vi "Problem 12 - Highly divisible triangular number.vi"(8 "error in (no error)":errorcluster) -> (0 "error out":errorcluster, 3 "Answer":u64)   [LabVIEW 2021, in "Project Euler.lvlib"]
uses:
  Project Euler.lvlib
  Utilities/Named Timers/Named Timers.lvlib
  Utilities/Numeric Utilities/Numeric Utilities.lvlib
panel:
  out "Triangular numbers":i32[](array[numeric])
  out "index of max no. of divisors":i32
  out "iteration execution time vs. iteration":u32[](graph)
  out "iteration execution time (ms)":u32
  in  "Dev: Stop early":bool
  out "max no. of divisors":i32
  in  "min requested no of divisors":i32=500
  in  "n = generate this many terms":u32=100
  out "Loop iteration":i32
  out "Total execution time (ms)":u32
  # "Development\ncontrols/indicators useful for development and testing, but which are not outputs of the VI"
  # "Input\nInputs to the VI"
  # "Output\nOutputs of the VI"
  # "Description\n\nBlank VI with error handling case. \n\nSummarize the use of this VI in this space."
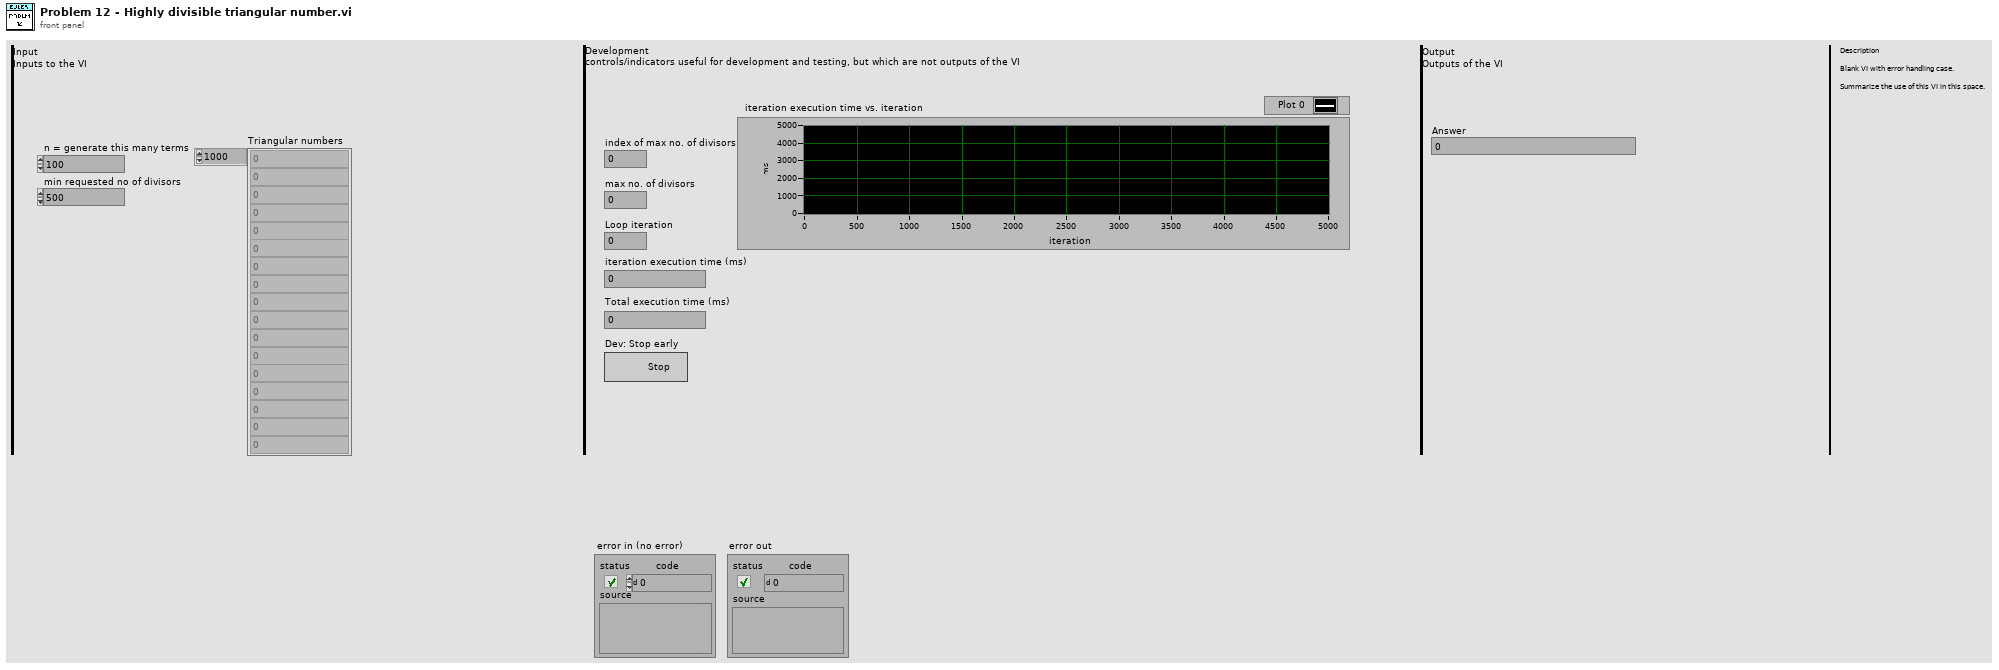
[diagram p1: front panel]
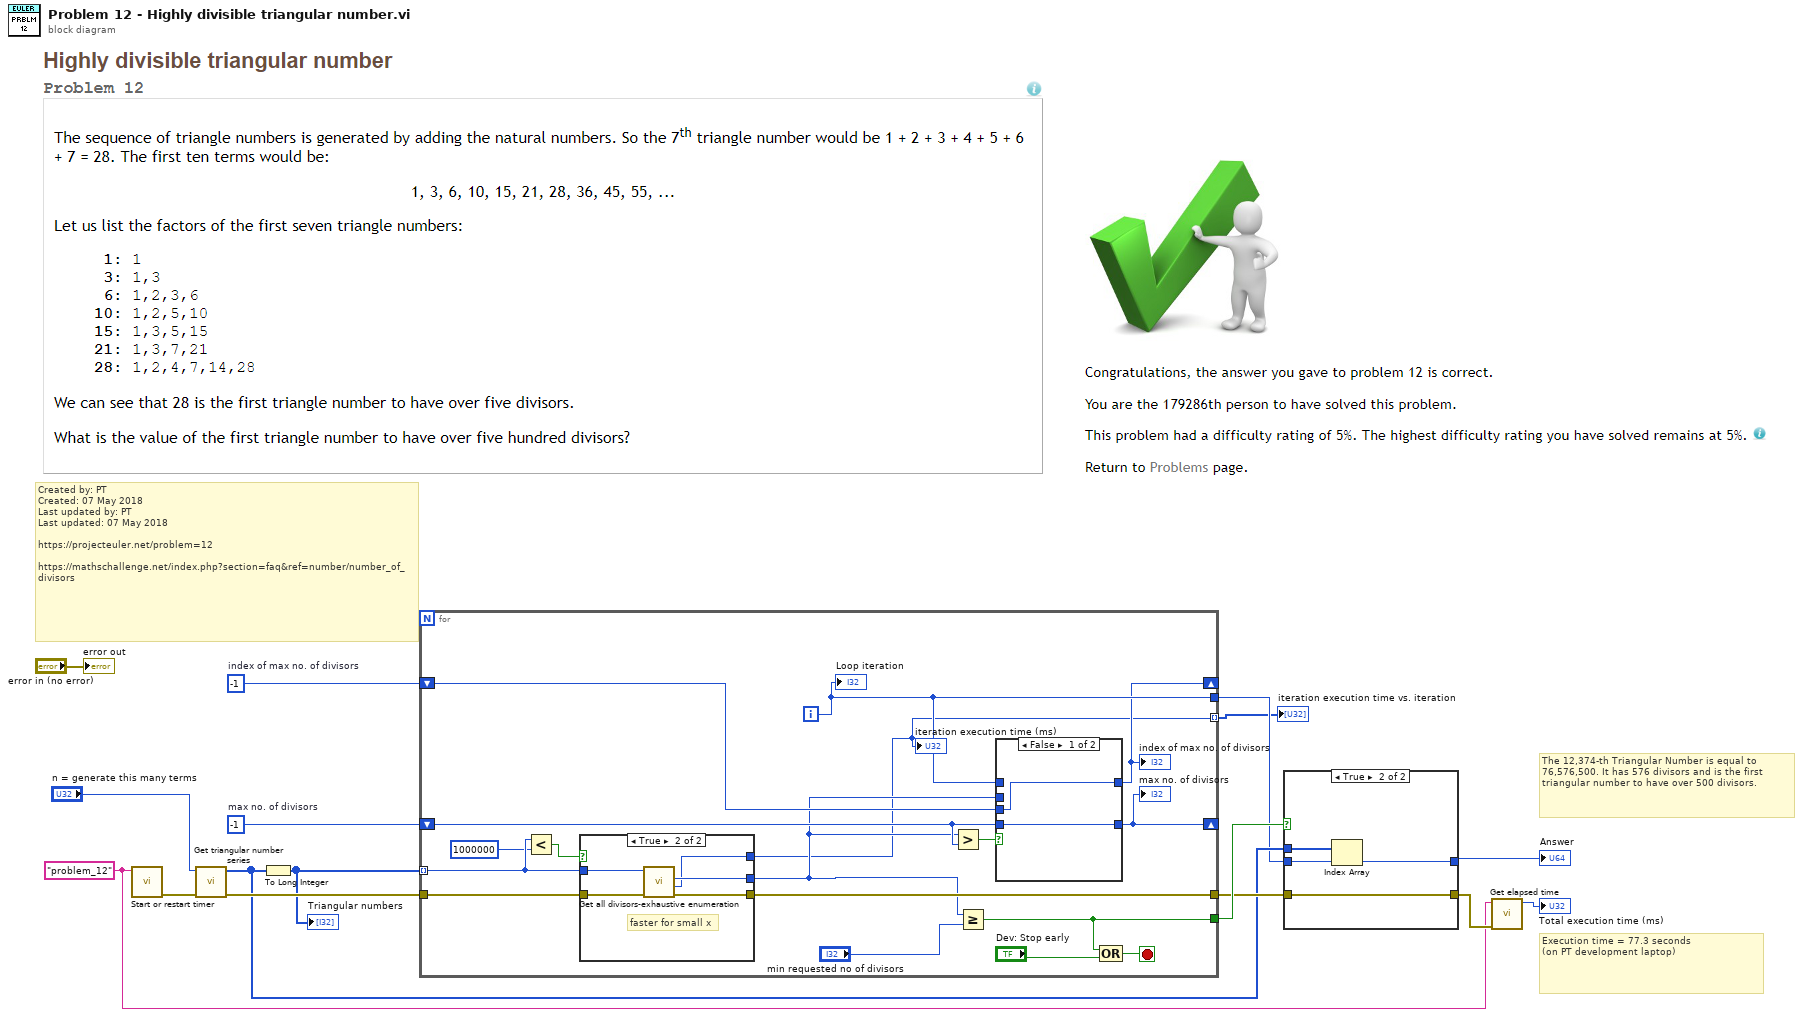
[diagram p0: block diagram]
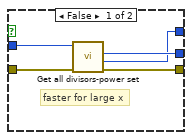
[diagram p3: hidden frame]
diagram:
  w1 = -1  # index of max no. of divisors
  w11 = -1  # max no. of divisors
  w4 = "problem_12" ("Timer name")
  # "The 12,374-th Triangular Number is equal to 76,576,500. It has 576 divisors and is the first triangular number to have over 500 divisors."
  # "Execution time = 77.3 seconds\n(on PT development laptop)"
  # "Created by: PT\nCreated: 07 May 2018\nLast updated by: PT\nLast updated: 07 May 2018\n\nhttps://projecteuler.net/problem=12\n\nhttps://mathschallenge.net/index.php?section=faq&ref=number/number_of_divisors"
  n1 = call "Start or restart timer.vi"("Timer name"=w4) -> ("error out"=w12:errorcluster)  [unwired: 10 in]
  n2 = call "Get triangular number series.vi"("error in (no error)"=w12, "n = generate this many terms (dflt=100)"="n = generate this many terms") -> ("error out"=w14:errorcluster, "Triangular numbers"=w8:u64[])  [unwired: 8 in]
  n3 = To Long Integer(number=w8) -> (32bit integer=w13:i32[])
  "Triangular numbers" <- w13
  n4 = for {
    tunnel: w14 -> [w33]
    tunnel: w13 -> [w21] mode=indexing
    tunnel: [w32] -> w9
    shift-right: [w28] -> _
    shift-left: w11 -> [w30]
    tunnel: [w24] -> w7
    tunnel: [w27] -> w10
    tunnel: [w18] -> w2 mode=indexing
    shift-right: [w23] -> _
    shift-left: w1 -> [w22]
    i -> [w24]
    stop <- w25 stop-if-true
    n5 = Less?(x=w21, y=1000000) -> (x < y?=w17:bool)
    n6 = case shown="True" w17 {
      tunnel: [w37 w43] -> w32
      tunnel: w33 -> [w38 w42]
      tunnel: w21 -> [w36 w41]
      tunnel: [w35 w40] -> w19
      tunnel: [w34 w39] -> w18
      frame False {
        # "faster for large x"
        n7 = call "Get all divisors-power set.vi"("error in (no error)"=w38, "x"=w36) -> ("error out"=w37:errorcluster, "Execution time (ms)-Total"=w34:u32, "no. of divisors"=w35:i32)  [unwired: 6 in, 1 out]
      }
      frame True {
        # "faster for small x"
        n8 = call "Get all divisors-exhaustive enumeration.vi"("error in (no error)"=w42, "x"=w41) -> ("error out"=w43:errorcluster, "Execution time (ms)-Total"=w39:u32, "no. of divisors"=w40:i32)  [unwired: 6 in, 1 out]
      }
    }
    "iteration execution time (ms)" <- w18
    n9 = Greater?(x=w19, y=w30) -> (0:w31:bool)
    n10 = Greater Or Equal?(x=w19, y="min requested no of divisors") -> (x >= y?=w27:bool)
    n11 = case shown="False" w31 {
      tunnel: [w45 w47] -> w28
      tunnel: w19 -> [_ w47]
      tunnel: w30 -> [w45 _]
      tunnel: w24 -> [_ w46]
      tunnel: [w44 w46] -> w23
      tunnel: w22 -> [w44 _]
      frame False {
      }
      frame True {
        # "new max"
      }
    }
    "max no. of divisors" <- w28
    "index of max no. of divisors" <- w23
    n12 = Compound Arithmetic op=OR(w27, "Dev: Stop early") -> (w25:bool)
    "Loop iteration" <- w24
  }
  "iteration execution time vs. iteration" <- w2
  n13 = case shown="True" w10 {
    tunnel: w9 -> [w48 w49]
    tunnel: w8 -> [_ w52]
    tunnel: w7 -> [_ w51]
    tunnel: [_ w50] -> w6
    tunnel: [w48 w49] -> w5
    frame False {
    }
    frame True {
      n14 = Index Array(array=w52, index=w51) -> (element=w50:u64)
    }
  }
  "Answer" <- w6
  n15 = call "Get elapsed time.vi"("error in (no error)"=w5, "Timer name"=w4) -> ("Elapsed time (ms)"=→"Total execution time (ms)":u32)  [unwired: 6 in, 3 out]
  "error out" <- "error in (no error)"
